vi "REACTOR_GLOBALES.vi"() -> ()   [LabVIEW 2017]
uses:
  REACTOR_COMUNICACIONES.ctl
  SERIAL ALICATS/__s_SPali4.ctl
  SERIAL ALICATS/__s_TablaAlicats.ctl
  EUROTHERM/TEG P116x2.ctl
  EUROTHERM/2xP116.ctl
panel:
  in  "stop":bool
  out "tPlato(s)":dbl format="%.1f"
  in  "P116x2":T1
  in  "VALVULA":bool
  out "ALICATS_RNG":T3
  out "T.Wait Stability":bool
  out "Mide Alicats":bool=TRUE
  out "Mide Temps":bool=TRUE
  out "ALICATS":T4=[["A", "NO", "aM0000013", "Air", "100", "ln/mn", "0.1", "0.11"], ["B", "NO", "aM0000014", "Air", "100", "ln/mn", "0.2", "0.22"], ["C", "NO", "aM0000015", "Air", "100", "ln/mn", "0.3", "0.33"], ["D", "NO", "aM0000016", "Air", "500", "ln/mn", "0.4", "0.44"]] caption="Alicats"
  in  "CAMBIO VAL":bool
  in  "CAMBIO TEMP":bool
  in  "CAMBIO ALIC":bool
  out "ALICATS_SP":T3
  in  "Comments":string
  out "Muestreo(s)":dbl format="%.1f"
  out "Max_t (s)":dbl format="%.1f"
  out "Delta_t (s)":dbl format="%.1f"
  out "Delta_T (C)":dbl format="%.1f"
  in  "T ESTABLE?":bool
  out "COMMS":T5={"Alicats"="ASRL6::INSTR", "Alic"=FALSE, "eValve"="ASRL6::INSTR", "eval"=FALSE, "Eurotherm"="ASRL6::INSTR", "euro"=FALSE, "Cell GAS"="ASRL6::INSTR", "cgas"=FALSE, "Cell H2S"="ASRL6::INSTR", "ch2s"=FALSE}
  in  "SALTAR":bool
  in  "PAUSA":bool
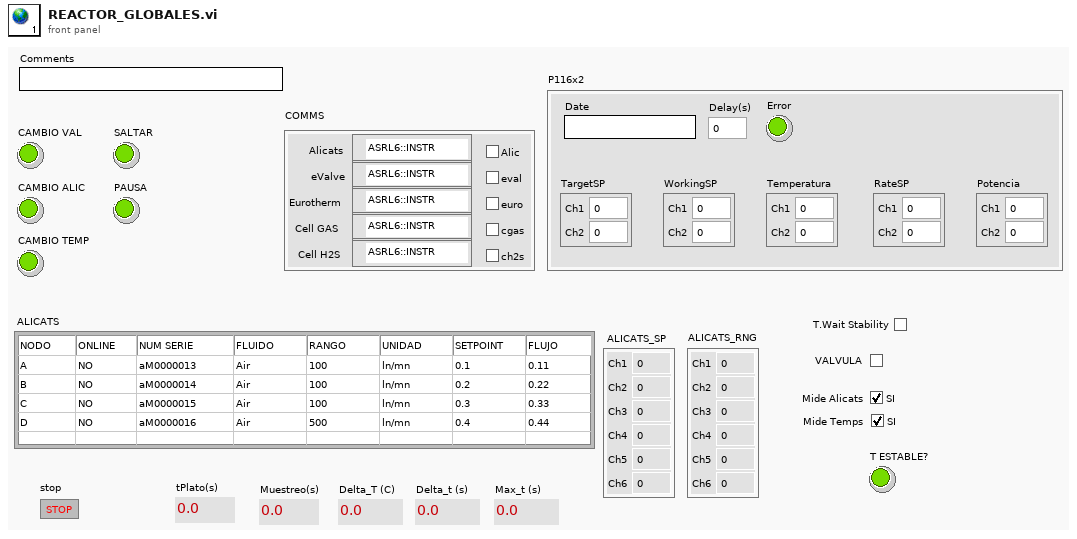
[diagram p1: front panel]
types:
  T1 = typedef "TEG P116x2.ctl" = cluster{"TargetSP":T2, "WorkingSP":T2, "Temperatura":T2, "Error":bool, "Date":string, "Delay(s)":dbl, "RateSP":T2, "Potencia":T2}
  T2 = typedef "2xP116.ctl" = cluster{"Ch1":dbl, "Ch2":dbl}
  T3 = typedef "__s_SPali4.ctl" = cluster{"Ch1":dbl, "Ch2":dbl, "Ch3":dbl, "Ch4":dbl, "Ch5":dbl, "Ch6":dbl}
  T4 = typedef "__s_TablaAlicats.ctl" = string[][]
  T5 = typedef "REACTOR_COMUNICACIONES.ctl" = cluster{"Alicats":refnum<visa-resource-name>, "Alic":bool, "eValve":refnum<visa-resource-name>, "eval":bool, "Eurotherm":refnum<visa-resource-name>, "euro":bool, "Cell GAS":refnum<visa-resource-name>, "cgas":bool, "Cell H2S":refnum<visa-resource-name>, "ch2s":bool}
diagram:
